vi "osa_globals.vi"() -> ()   [LabVIEW 2021]
panel:
  out "stop osa panel...":bool
  out "measuring...":bool
  # "odor sensor array: global variables for control"
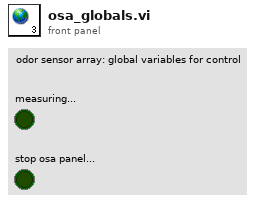
[diagram p1: front panel]
diagram:
